vi "Enumprog.vi"() -> ()   [LabVIEW 2019]
panel:
  out "Month":T1(ring)
  out "Weekday":T2(ring)
  in  "month":T1(ring)
  in  "weekday":T2(ring)
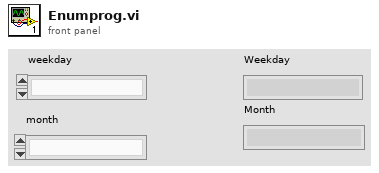
[diagram p1: front panel]
types:
  T1 = enum16{"", "January", "February", "March", "April", "May", "June", "July", "August", "September", "October", "November", "December"}
  T2 = enum16{"", "Monday", "Tuesday", "Wednesday", "Thrusday", "Friday", "Saturday", "Sunday"}
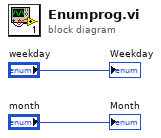
[diagram p0: block diagram]
diagram:
  "Weekday" <- "weekday"
  "Month" <- "month"
